vi "lab4.vi"() -> ()   [LabVIEW 2020]
panel:
  out "XY Graph":cluster{"Y":dbl[], "Y":dbl[]}[](graph)
  out "Array 2":dbl[][](array[numeric])
  out "Array":dbl[][](array[numeric])
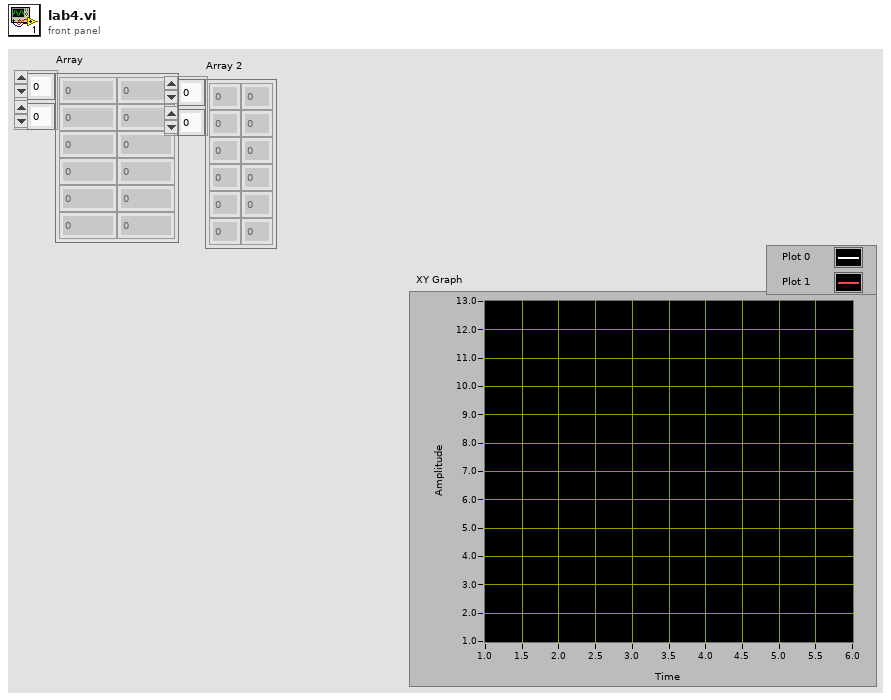
[diagram p1: front panel]
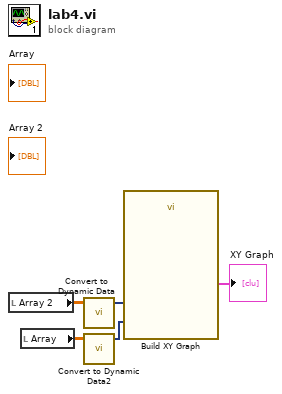
[diagram p0: block diagram]
diagram:
  n1 = local read "Array 2"() -> (w4:dbl[][])
  n2 = local read "Array"() -> (w2:dbl[][])
  n3 = call "Convert to Dynamic Data"("2D Array"=w4) -> ("Dynamic Data Type"=w3:dynamicdata)  [unwired: 3 in]
  n4 = call "Convert to Dynamic Data2"("2D Array"=w2) -> ("Dynamic Data Type"=w1:dynamicdata)  [unwired: 3 in]
  n5 = call "Build XY Graph"("Y Input"=w3, "X Input"=w1) -> ("XY Graph"=→"XY Graph":cluster{"X":dbl[], "Y":dbl[]}[])  [unwired: 8 in, 1 out]
